vi "Low Pass Differentiator.vi"   [LabVIEW 2011]
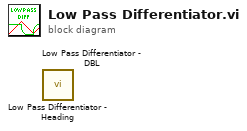
[diagram p0: block diagram]
diagram:
  n1 = call "Low Pass Differentiator - Heading.vi"() -> ()  [unwired: 11 in, 1 out]
  n2 = call "Low Pass Differentiator - DBL.vi"() -> ()  [unwired: 11 in, 1 out]
